vi "3_Ejes.vi"() -> ()   [LabVIEW 2017]
uses:
  <vilib>/Motion/Express/_s/nimc.fb.straightLineMove.startStraightLineMove.axis.modeAbsolute.0.vi
  <vilib>/Motion/Express/_s/nimc.fb.read.readExecutionData.axis.vi
  <vilib>/Motion/Express/_s/nimc.fb.contourMove.startContourMove.axis.modeFinite.vi
  <vilib>/Motion/BlockNode/FB.NIMotion.xnode
  <vilib>/Motion/Express/_s/nimc.fb.contourMove.splineType.ctl
panel:
  in  "Play Button":bool
  out "Eje x":dbl(slide) scale=-100.0..100.0
  out "Exje Y":dbl(slide)=-0.0 scale=-100.0..100.0
  out "XY Graph":cluster{dbl[], dbl[]}(graph)
  in  "Stop Button":bool
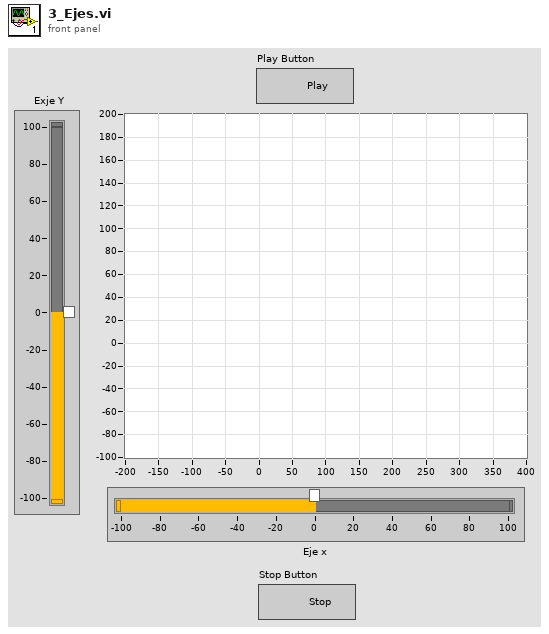
[diagram p1: front panel]
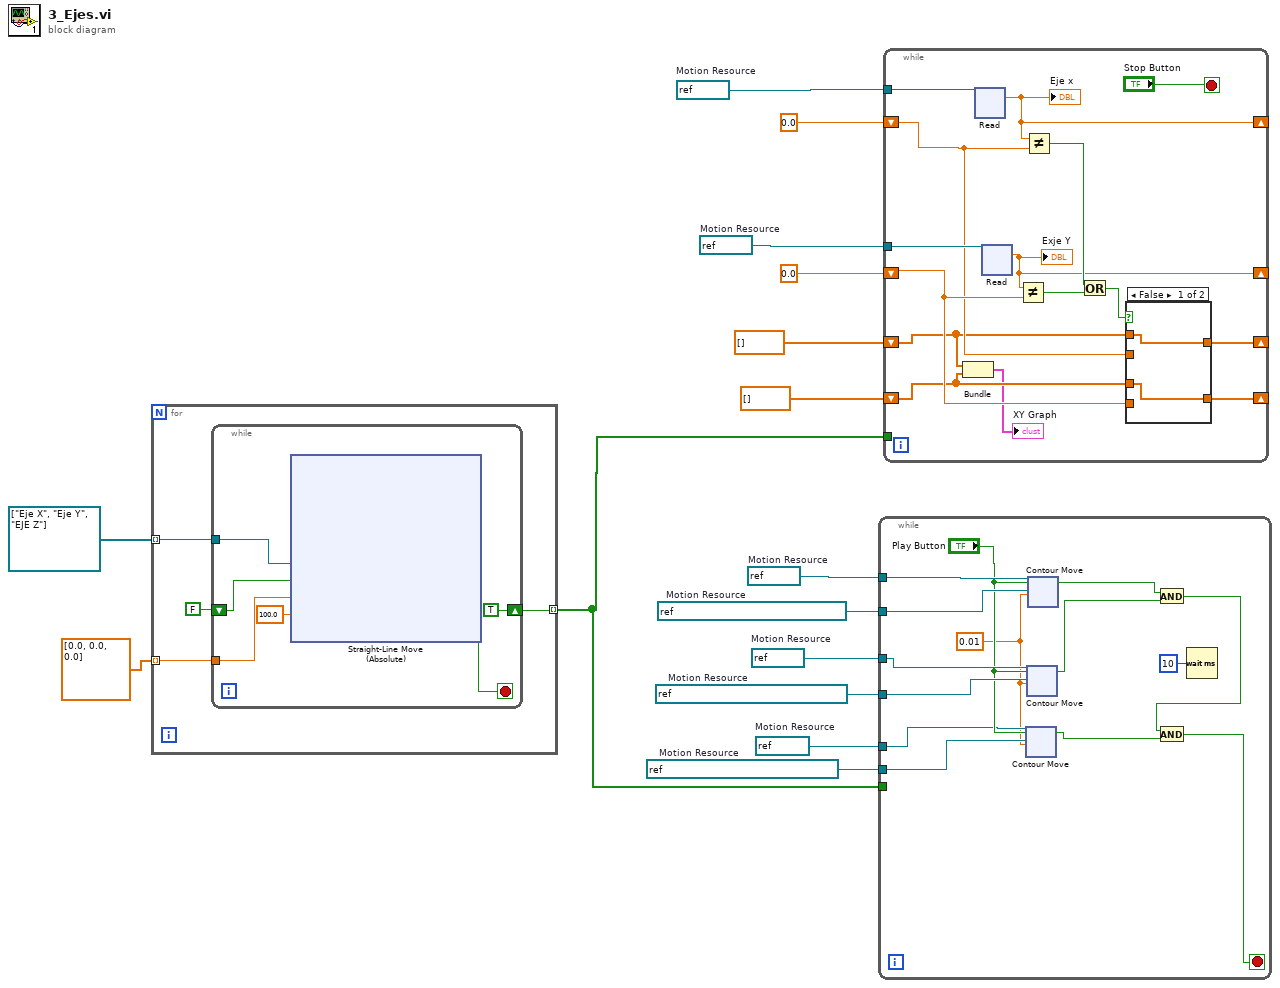
[diagram p0: block diagram]
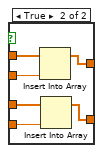
[diagram p2: hidden frame]
diagram:
  w1 = refnum<k21> "TablaY"  # Motion Resource
  w2 = refnum<k21> "EJE Z"  # Motion Resource
  w5 = refnum<k21> "TablaX"  # Motion Resource
  w4 = refnum<k21> "TablaY"  # Motion Resource
  w6 = refnum<k21> "Eje Y"  # Motion Resource
  w7 = refnum<k21> "Eje X"  # Motion Resource
  w14 = refnum<k21> "Eje Y"  # Motion Resource
  w15 = refnum<k21> "Eje X"  # Motion Resource
  n1 = for {
    tunnel: refnum<k21>[] ["Eje X", "Eje Y", "EJE Z"] -> [w17] mode=indexing
    tunnel: dbl[] [0.0, 0.0, 0.0] -> [w18] mode=indexing
    tunnel: [w16] -> w3 mode=indexing
    n2 = while {
      shift-right: [TRUE] -> w16
      shift-left: FALSE -> [w25]
      tunnel: w18 -> [w22]
      tunnel: w17 -> [w21]
      stop <- w24 stop-if-true
      n3 = xnode "Straight-Line Move\n(Absolute)"("resource"=w21, "execute"=w25, "position"=w22, "velocity"=100.0) -> ("done"=w24:bool)  [unwired: 2 in, 2 out]
    }
  }
  n4 = while {
    tunnel: w7 -> [w56]
    tunnel: w6 -> [w54]
    tunnel: w5 -> [w53]
    tunnel: w4 -> [w52]
    tunnel: w3 -> [_]
    tunnel: w2 -> [w44]
    tunnel: w1 -> [w46]
    stop <- w47 stop-if-true
    w43 = 0.01 ("interval")
    n5 = xnode "Contour Move"("resource"=w44, "execute"="Play Button", "table"=w46, "interval"=w43) -> ("done"=w49:bool)  [unwired: 2 in, 5 out]
    n6 = xnode "Contour Move"("resource"=w54, "execute"="Play Button", "table"=w52, "interval"=w43) -> ("done"=w51:bool)  [unwired: 2 in, 5 out]
    n7 = xnode "Contour Move"("resource"=w56, "execute"="Play Button", "table"=w53, "interval"=w43) -> ("done"=w55:bool)  [unwired: 2 in, 5 out]
    n8 = And(x=w55, y=w51) -> (x .and. y?=w48:bool)
    n9 = And(x=w48, y=w49) -> (x .and. y?=w47:bool)
    n10 = Wait (ms)(milliseconds to wait=u32 10) -> ()  [unwired: 1 out]
  }
  n11 = while {
    tunnel: w15 -> [w137]
    tunnel: w14 -> [w136]
    shift-right: [w125] -> _
    shift-left: 0.0 ("position") -> [w129]
    shift-right: [w124] -> _
    shift-left: 0.0 ("position") -> [w130]
    shift-right: [w132] -> _
    shift-left: dbl[] [] -> [w128]
    shift-right: [w131] -> _
    shift-left: dbl[] [] -> [w127]
    tunnel: w3 -> [_]
    stop <- "Stop Button" stop-if-true
    n12 = Bundle(w128, w127) -> (→"XY Graph":cluster{dbl[], dbl[]})  [unwired: 1 in]
    n13 = xnode "Read"("resource"=w137) -> ("position"=w125:dbl)  [unwired: 2 in, 7 out]
    "Eje x" <- w125
    n14 = xnode "Read"("resource"=w136) -> ("position"=w124:dbl)  [unwired: 2 in, 7 out]
    "Exje Y" <- w124
    n15 = Not Equal?(x=w124, y=w130) -> (x != y?=w134:bool)
    n16 = Not Equal?(x=w125, y=w129) -> (x != y?=w135:bool)
    n17 = Or(x=w135, y=w134) -> (x .or. y?=w133:bool)
    n18 = case shown="False" w133 {
      tunnel: w128 -> [w139 w145]
      tunnel: [w139 w144] -> w132
      tunnel: w127 -> [w138 w143]
      tunnel: [w138 w142] -> w131
      tunnel: w130 -> [_ w141]
      tunnel: w129 -> [_ w140]
      frame False {
      }
      frame True {
        n19 = Insert Into Array(array=w145, new element=w140) -> (w144:dbl[])  [unwired: 1 in]
        n20 = Insert Into Array(array=w143, new element=w141) -> (w142:dbl[])  [unwired: 1 in]
      }
    }
  }
